vi "Read panel mode.vi"(8 "error in (no error)":errorcluster, 11 "RocketPlotPanel in":refnum<class "RocketPlotPanel.lvclass">) -> (0 "error out":errorcluster, 2 "Enum":T1, 3 "RocketPlotPanel out":refnum<class "RocketPlotPanel.lvclass">)   [LabVIEW 2021, in "RocketPlot.lvlib" / "RocketPlotPanel.lvclass"]
uses:
  RocketPlotPanel.lvclass
  RocketPlotPanel.lvclass/RocketPlotPanel.ctl
  TypeDefs/panel mode.ctl
  RocketPlot.lvlib
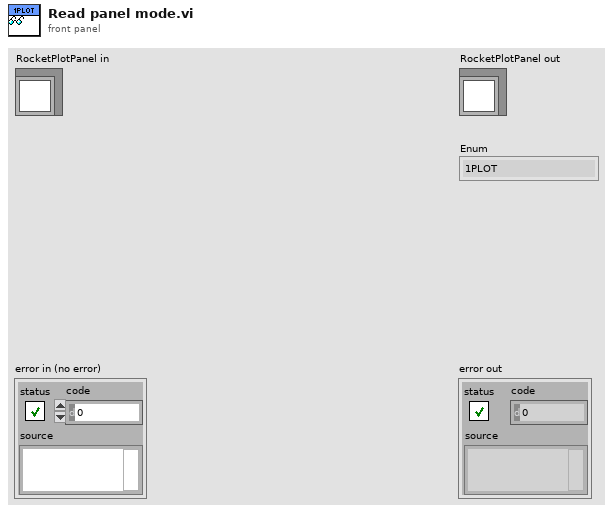
[diagram p1: front panel]
types:
  T1 = typedef "RocketPlot.lvlib/panel mode.ctl" = enum16{"1PLOT", "MPLOT"}
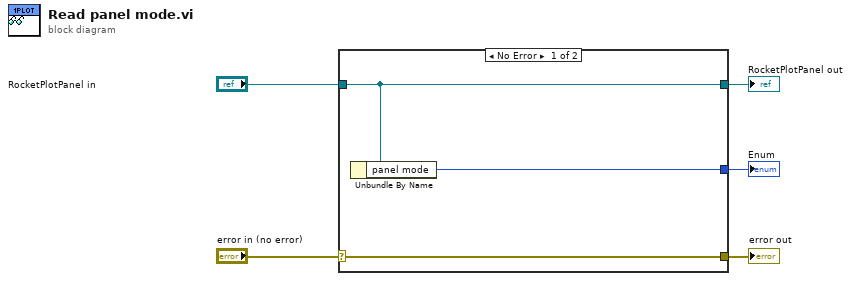
[diagram p0: block diagram]
diagram:
  n1 = case shown="No Error" "error in (no error)" {
    selector: "error in (no error)" -> [w8 w9]
    tunnel: [w8 w9] -> w4
    tunnel: [w7 w10] -> w2
    tunnel: "RocketPlotPanel in" -> [w7 w10]
    tunnel: [w6 _] -> w1
    frame No Error {
      n2 = Unbundle By Name(w7) -> ("panel mode"=w6:T1)
    }
    frame Error {
    }
  }
  "error out" <- w4
  "RocketPlotPanel out" <- w2
  "Enum" <- w1
